vi "xijk_save_search_xijk_to_file.vi"(5 "filepaths in":T3, 7 "search paths in":T2, 8 "error in":errorcluster, 11 "output cluster":T1) -> (0 "error out":errorcluster)   [LabVIEW 2009]
uses:
  Type Def/filepath.ctl
  Type Def/search_parameters.ctl
  Type Def/xijk_cluster.ctl
  <vilib>/Utility/file.llb/Write To Spreadsheet File (string).vi
  xijk_select_best_filter.lvlib
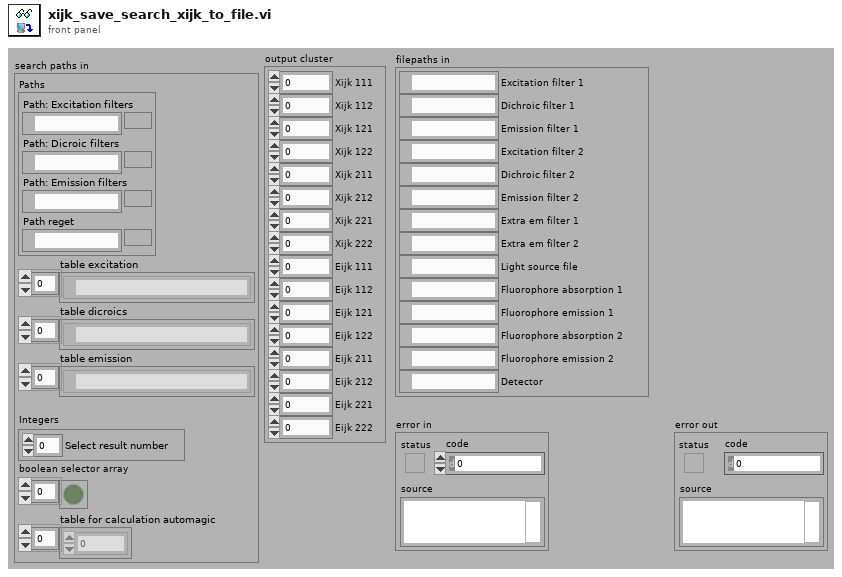
[diagram p1: front panel]
types:
  T1 = typedef "xijk_cluster.ctl" = cluster{"Xijk 111":sgl, "Xijk 112":sgl, "Xijk 121":sgl, "Xijk 122":sgl, "Xijk 211":sgl, "Xijk 212":sgl, "Xijk 221":sgl, "Xijk 222":sgl, "Eijk 111":sgl, "Eijk 112":sgl, "Eijk 121":sgl, "Eijk 122":sgl, "Eijk 211":sgl, "Eijk 212":sgl, "Eijk 221":sgl, "Eijk 222":sgl}
  T2 = typedef "search_parameters.ctl" = cluster{"Paths":cluster{"Path: Excitation filters":path, "Path: Dicroic filters":path, "Path: Emission filters":path, "Path reget":path}, "table excitation":path[], "table dicroics":path[], "table emission":path[], "Integers":cluster{"Select result number":u32}, "boolean selector array":bool[], "table for calculation automagic":i32[]}
  T3 = typedef "filepath.ctl" = cluster{"Excitation filter 1":path, "Dichroic filter 1":path, "Emission filter 1":path, "Excitation filter 2":path, "Dichroic filter 2":path, "Emission filter 2":path, "Extra em filter 1":path, "Extra em filter 2":path, "Light source file":path, "Fluorophore absorption 1":path, "Fluorophore emission 1":path, "Fluorophore absorption 2":path, "Fluorophore emission 2":path, "Detector":path}
  T4 = cluster{"Excitation filter 1":string, "Dichroic filter 1":string, "Emission filter 1":string, "Excitation filter 2":string, "Dichroic filter 2":string, "Emission filter 2":string, "Extra em filter 1":string, "Extra em filter 2":string, "Light source file":string, "Fluorophore absorption 1":string, "Fluorophore emission 1":string, "Fluorophore absorption 2":string, "Fluorophore emission 2":string, "Detector":string}
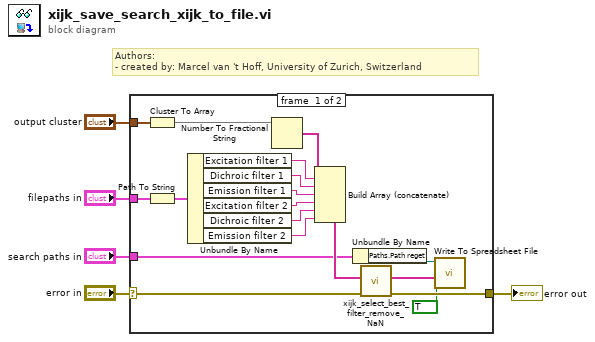
[diagram p0: block diagram]
diagram:
  # "Authors: \n- created by: Marcel van 't Hoff, University of Zurich, Switzerland"
  n1 = case shown="No Error" "error in" {
    selector: "error in" -> [w6 w24]
    tunnel: "filepaths in" -> [w14 _]
    tunnel: [w13 w24] -> w4
    tunnel: "search paths in" -> [w11 _]
    tunnel: "output cluster" -> [w7 _]
    frame #0 {
      n2 = Cluster To Array(cluster=w7) -> (array=w8:sgl[])
      n3 = Path To String(path=w14) -> (string=w15:T4)
      n4 = Unbundle By Name(w15) -> ("Excitation filter 1"=w17:string, "Dichroic filter 1"=w18:string, "Emission filter 1"=w19:string, "Excitation filter 2"=w20:string, "Dichroic filter 2"=w21:string, "Emission filter 2"=w22:string)
      n5 = Number To Fractional String(number=w8) -> (F-format string=w16:string[])  [unwired: 3 in]
      n6 = Build Array (concatenate)(w16, w17, w18, w19, w20, w21, w22) -> (w23:string[])
      n7 = Unbundle By Name(w11) -> ("Paths.Path reget"=w12:path)
      n8 = call "xijk_select_best_filter_remove_NaN.vi"("error in"=w6, "table_input_1D"=w23) -> ("error out"=w13:errorcluster, "table_output_1D"=w10:string[])  [unwired: 7 in, 1 out]
      n9 = call-poly <vilib>:"Write To Spreadsheet File.vi"("append to file? (new file:F)"=TRUE, "1D data"=w10, "file path (dialog if empty)"=w12) -> ()  [unwired: 3 in, 3 out]
    }
    frame #1 {
    }
  }
  "error out" <- w4
